vi "Pre Launch Init.vi"(11 "UI_Actor in":refnum<class "UI_Actor.lvclass">) -> (0 "error out":errorcluster, 3 "UI_Actor out":refnum<class "UI_Actor.lvclass">)   [LabVIEW 2020, in "UI_Actor.lvlib" / "UI_Actor.lvclass"]
doc: "(<B>Filename</B>: Actor Framework.lvlib:Actor.lvclass:Pre Launch Init.vi)\n\nDefines behavior that occurs after the Launch Nested Actor method is invoked but before the actor's Actor Core method begins running.\n\nBy default, this method does nothing. A descendant class may override it to define behavior."
uses:
  UI_Actor.lvclass
  ctl_UE_Msg.ctl
  UI_Actor.lvclass/UI_Actor.ctl
  ctl_InternalMapItem.ctl
  support/Databox.lvlibp/TypesTools/Config/Config.lvclass
  support/Databox.lvlibp/TypesTools/Data/Data.lvclass
  support/Actor Framework.lvlibp/1abvi3w/vi.lib/ActorFramework/Actor/Actor.lvclass
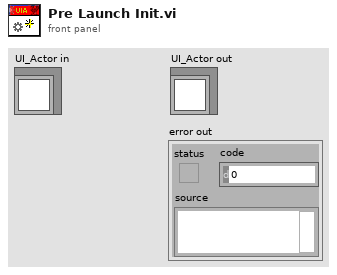
[diagram p1: front panel]
types:
  T1 = typedef "UI_Actor.lvlib/UI_Actor.lvclass/ctl_UE_Msg.ctl" = cluster{"Cmd":string, "Payload":string}
  T2 = typedef "UI_Actor.lvlib/UI_Actor.lvclass/ctl_InternalMapItem.ctl" = cluster{"Config":refnum<class "Config.lvclass">, "LatestData":refnum<class "Data.lvclass">}
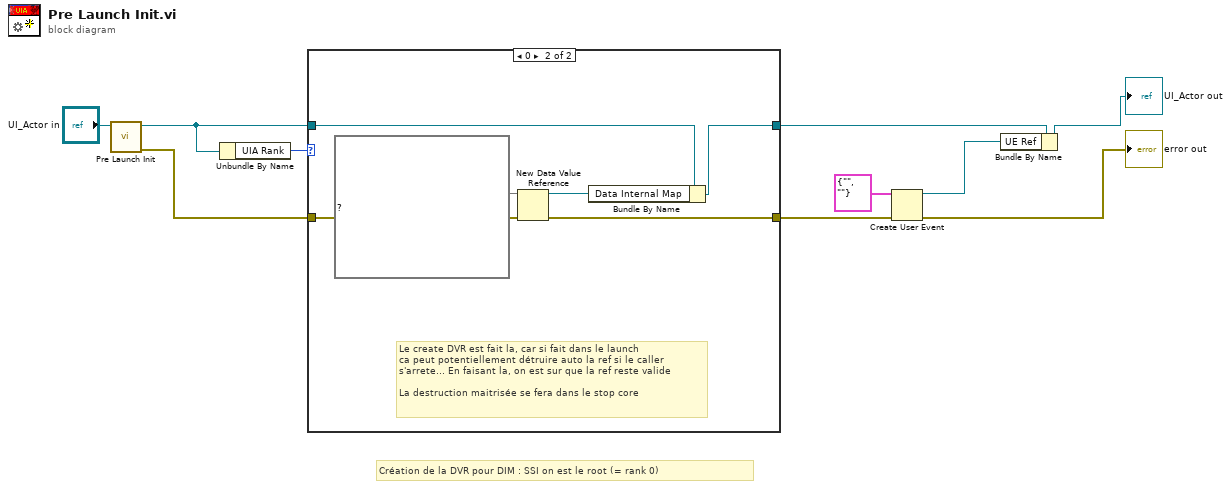
[diagram p0: block diagram]
diagram:
  # "Création de la DVR pour DIM : SSI on est le root (= rank 0)"
  n1 = call-parent "Pre Launch Init.vi"("Actor in"="UI_Actor in") -> ("error out"=w6:errorcluster, "Actor out"=w8:refnum<class "UI_Actor.lvclass">)  [unwired: 9 in]
  n2 = Unbundle By Name(w8) -> ("UIA Rank"=w9:i32)
  n3 = case shown="0" w9 {
    tunnel: [w12 w18] -> w7
    tunnel: w6 -> [w11 w17]
    tunnel: [w11 w16] -> w1
    tunnel: w8 -> [w12 w15]
    frame Default {
    }
    frame 0 {
      # "Le create DVR est fait la, car si fait dans le launch\nca peut potentiellement détruire auto la ref si le caller\ns'arrete... En faisant la, on est sur que la ref reste valide\n\nLa destruction maitrisée se fera dans le stop core"
      n4 = New Data Value Reference(data value=map{string, map{string, T2}} {} ("Map"), error in=w17) -> (data value reference=w14:refnum<data-value>, error out=w16:errorcluster)
      n5 = Bundle By Name(cluster=w15, "Data Internal Map"=w14) -> (w18:refnum<class "UI_Actor.lvclass">)
    }
  }
  n6 = Create User Event(user event datatype=T1 {"Cmd"="", "Payload"=""} ("UE_Msg"), error in=w1) -> (user event=w3:refnum<user-event>, error out=→"error out":errorcluster)
  n7 = Bundle By Name(cluster=w7, "UE Ref"=w3) -> (→"UI_Actor out":refnum<class "UI_Actor.lvclass">)
